vi "VIPM Pre-Build Custom Action.vi"(10 "Variant":variant) -> (0 "error out":errorcluster)   [LabVIEW 2020]
uses:
  dev/Tags.ctl
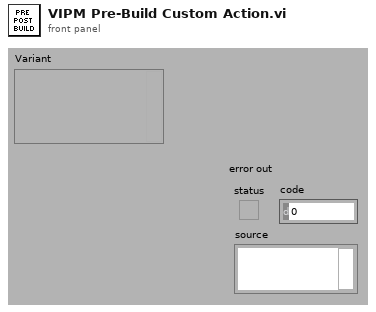
[diagram p1: front panel]
types:
  T1 = typedef "Tags.ctl" = enum16{"sol.squarebattle.version"}
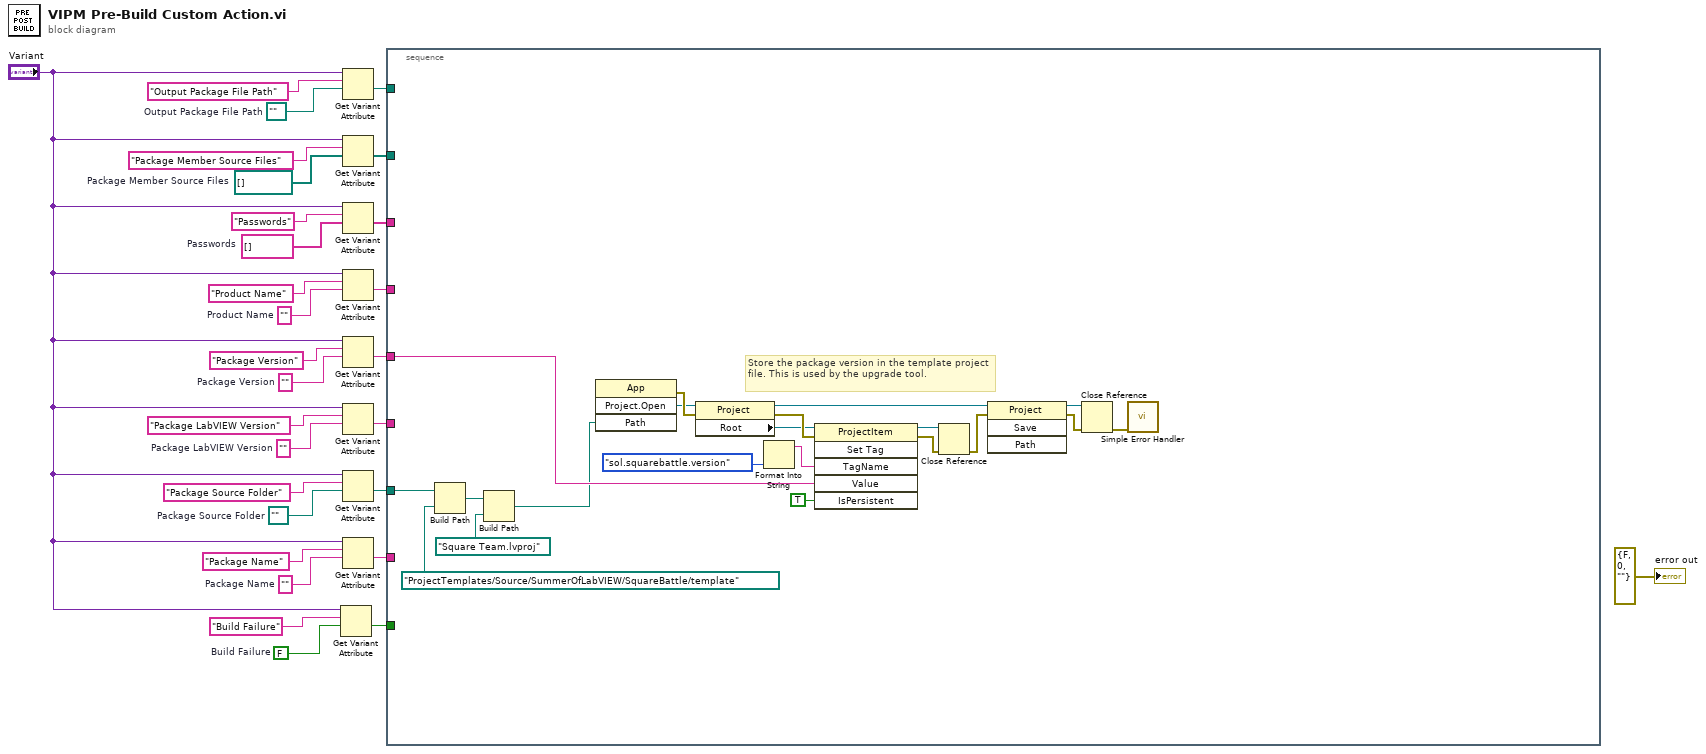
[diagram p0: block diagram]
diagram:
  w3 = FALSE  # Build Failure
  w13 = path ""  # Package Source Folder
  w14 = ""  # Package Name
  w17 = ""  # Package LabVIEW Version
  w19 = ""  # Package Version
  w21 = ""  # Product Name
  w24 = string[] []  # Passwords
  w26 = path[] []  # Package Member Source Files
  w28 = path ""  # Output Package File Path
  n1 = Get Variant Attribute(Variant="Variant", name="Build Failure", default value (empty Variant)=w3) -> (value=w1:bool)  [unwired: 1 in, 3 out]
  n2 = Get Variant Attribute(Variant="Variant", name="Output Package File Path", default value (empty Variant)=w28) -> (value=w12:path)  [unwired: 1 in, 3 out]
  n3 = Get Variant Attribute(Variant="Variant", name="Package Member Source Files", default value (empty Variant)=w26) -> (value=w11:path[])  [unwired: 1 in, 3 out]
  n4 = Get Variant Attribute(Variant="Variant", name="Passwords", default value (empty Variant)=w24) -> (value=w10:string[])  [unwired: 1 in, 3 out]
  n5 = Get Variant Attribute(Variant="Variant", name="Product Name", default value (empty Variant)=w21) -> (value=w9:string)  [unwired: 1 in, 3 out]
  n6 = Get Variant Attribute(Variant="Variant", name="Package Version", default value (empty Variant)=w19) -> (value=w8:string)  [unwired: 1 in, 3 out]
  n7 = Get Variant Attribute(Variant="Variant", name="Package LabVIEW Version", default value (empty Variant)=w17) -> (value=w7:string)  [unwired: 1 in, 3 out]
  n8 = Get Variant Attribute(Variant="Variant", name="Package Source Folder", default value (empty Variant)=w13) -> (value=w6:path)  [unwired: 1 in, 3 out]
  n9 = Get Variant Attribute(Variant="Variant", name="Package Name", default value (empty Variant)=w14) -> (value=w5:string)  [unwired: 1 in, 3 out]
  n10 = stacked-sequence {
    tunnel: w12 -> [_]
    tunnel: w11 -> [_]
    tunnel: w10 -> [_]
    tunnel: w9 -> [_]
    tunnel: w8 -> [w40]
    tunnel: w7 -> [_]
    tunnel: w6 -> [w47]
    tunnel: w5 -> [_]
    tunnel: w1 -> [_]
    frame #0 {
      # "Store the package version in the template project file. This is used by the upgrade tool."
      n11 = Build Path(base path=w47, name or relative path=path "ProjectTemplates/Source/SummerOfLabVIEW/SquareBattle/template") -> (appended path=w45:path)
      n12 = Build Path(base path=w45, name or relative path=path "Square Team.lvproj") -> (appended path=w32:path)
      n13 = invoke class="App" method="Project.Open"("Path"=w32) -> (error out=w49:errorcluster, "Project:Open"=w42:refnum<vi>)  [unwired: 3 in, 2 out]
      n14 = property class="Project"(reference=w42, error in=w49) -> (reference out=w43:refnum<vi>, error out=w48:errorcluster, "Root"=w41:refnum<vi>)
      n15 = Format Into String(Tags."sol.squarebattle.version" ("Tags")) -> (resulting string=w30:string)  [unwired: 3 in, 1 out]
      n16 = invoke class="ProjectItem" method="Set Tag"(reference=w41, error in=w48, "TagName"=w30, "Value"=w40, "IsPersistent"=TRUE ("Is Persistent (T)")) -> (reference out=w38:refnum<vi>, error out=w37:errorcluster)  [unwired: 1 in, 4 out]
      n17 = Close Reference(reference=w38, error in (no error)=w37) -> (error out=w36:errorcluster)
      n18 = invoke class="Project" method="Save"(reference=w43, error in=w36) -> (reference out=w35:refnum<vi>, error out=w34:errorcluster)  [unwired: 2 in, 2 out]
      n19 = Close Reference(reference=w35, error in (no error)=w34) -> (error out=w33:errorcluster)
      n20 = call <vilib>:"Simple Error Handler.vi"("error in (no error)"=w33) -> ()  [unwired: 4 in, 5 out]
    }
  }
  "error out" <- errorcluster {"status"=FALSE, "code"=0, "source"=""} ("error out")
